vi "svx_Multitone Generator.vi"(5 "amplitude":dbl=-1.0 format="%.2f", 6 "sampling info":cluster{"Fs":dbl, "#s":dbl}={"Fs"=1000.0, "#s"=1000.0} {"#s" format="%.2p"; "Fs" format="%.2p"}, 8 "error in (no error)":errorcluster, 9 "tone phases":dbl[](array[numeric])=[137.63, 330.58, 66.37, 291.58, 225.38] format="%.2f", 10 "tone amplitudes":dbl[](array[numeric])=[1.0, 1.0, 1.0, 1.0, 1.0] format="%.2f", 11 "tone frequencies":dbl[](array[numeric])=[100.0, 200.0, 300.0, 400.0, 500.0] format="%.2f") -> (0 "error out":errorcluster, 2 "crest factor":dbl format="%.2f", 3 "signal out":waveform(dbl))   [LabVIEW 2017]
doc: "This VI generates a waveform that is the sum of integer cycle sine tones. The frequency domain representation of this waveform is a sequence of impulses at the specified tone frequencies and zero at all other frequencies. The number of tones is determined by the size of the array inputs (<B>tone frequencies</B>, <B>tone amplitudes</B>, and <B>phases</B>). First, the sine tones are generated using the frequency, phase, amplitude and samples information. This raw array is then scaled so that the largest absolute value is equal to the <B>amplitude</B> input. Finally the waveform is bundled. The X0 element of the waveform is always set equal to 0 and the delta X element is set equal to 1/(Sampling Rate)."
uses:
  <vilib>/Analysis/2dsp.llb/Inverse Real FFT.vi
  <vilib>/Analysis/5stat.llb/RMS (DBL).vi
  <vilib>/measure/NI_MABase.lvlib
  <vilib>/measure/NI_MAPro.lvlib
  <vilib>/Analysis/NI_AALPro.lvlib
  <vilib>/Analysis/NI_AALBase.lvlib
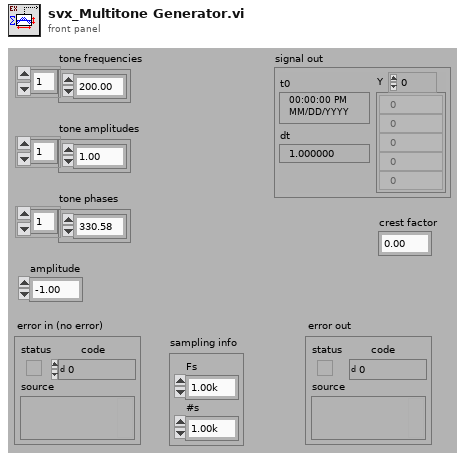
[diagram p1: front panel]
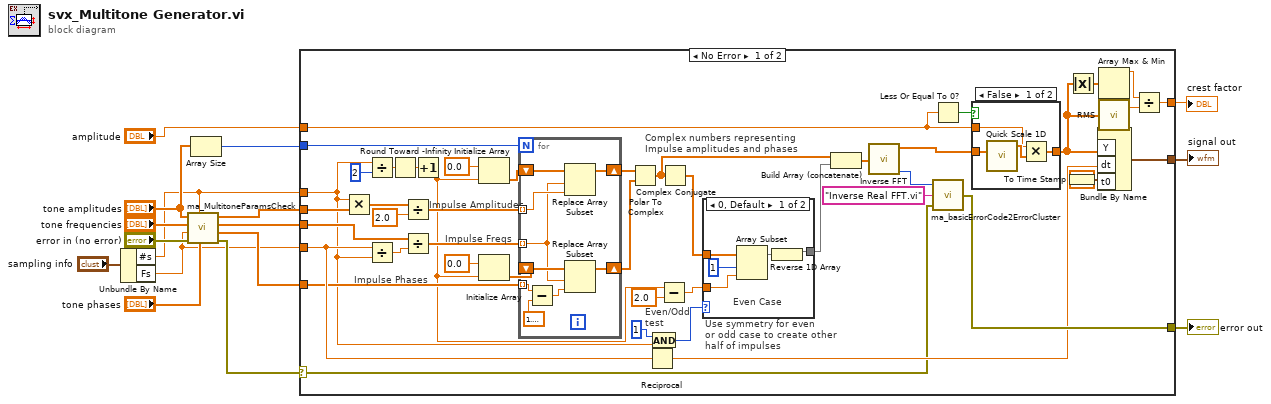
[diagram p0: block diagram]
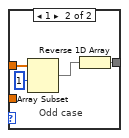
[diagram p3: hidden frame]
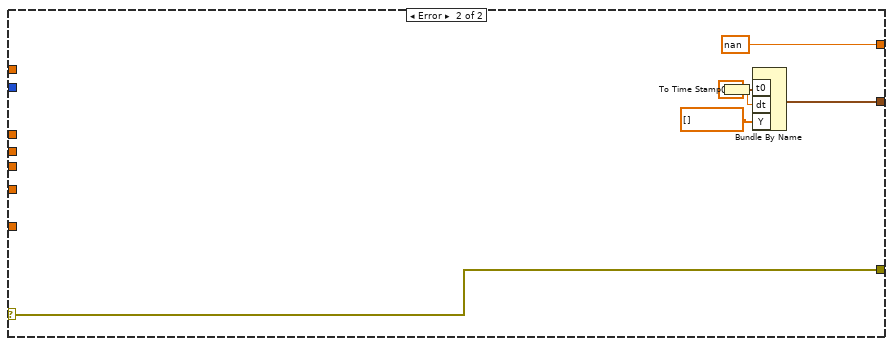
[diagram p4: hidden frame]
diagram:
  n1 = Unbundle By Name("sampling info") -> ("#s"=w4:dbl, "Fs"=w5:dbl)
  n2 = call <vilib>:"ma_MultitoneParamsCheck.vi"("Phases"="tone phases", "Samples"=w4, "error in (no error)"="error in (no error)", "Sampling Rate"=w5, "Tone Frequencies"="tone frequencies", "Tone Amplitudes"="tone amplitudes") -> ("error out"=w7:errorcluster, "Phases out"=w11:dbl[], "Tone Frequencies out"=w13:dbl[], "Tone Amplitudes out"=w8:dbl[])  [unwired: 2 in]
  n3 = Array Size(array="tone amplitudes") -> (size(s)=w15:i32)
  n4 = case shown="No Error" w7 {
    selector: w7 -> [w18 w86]
    tunnel: w5 -> [w59 _]
    tunnel: [w61 w86] -> w16
    tunnel: w15 -> [w60 _]
    tunnel: w4 -> [w32 _]
    tunnel: w13 -> [w58 _]
    tunnel: w11 -> [w37 _]
    tunnel: w8 -> [w36 _]
    tunnel: "amplitude" -> [w33 _]
    tunnel: [w25 nan] -> w2
    tunnel: [w24 w87] -> w1
    frame No Error {
      # "Impulse Phases"
      # "Use symmetry for even\nor odd case to create other\nhalf of impulses"
      # "Even/Odd\ntest"
      # "Complex numbers representing \nImpulse amplitudes and phases"
      # "Impulse Freqs"
      # "Impulse Amplitudes"
      n5 = Multiply(x=w32, y=w36) -> (x*y=w53:dbl[])
      n6 = Divide(x=w32, y=2) -> (x/y=w23:dbl)
      n7 = Divide(x=w59, y=w32) -> (x/y=w52:dbl)
      n8 = Round Toward -Infinity(1:w23) -> (0:w22:dbl)
      n9 = Divide(x=w53, y=2.0) -> (x/y=w55:dbl[])
      n10 = Divide(x=w58, y=w52) -> (x/y=w56:dbl[])
      n11 = Increment(x=w22) -> (x+1=w20:dbl)
      n12 = Initialize Array(0.0 ("Element Data"), w20) -> (w48:dbl[])
      n13 = Initialize Array(0.0 ("Element Data"), w20) -> (w47:dbl[])
      n14 = for {
        N: w60 -> [_]
        tunnel: w56 -> [w79] mode=indexing
        tunnel: w55 -> [w84] mode=indexing
        shift-right: [w82] -> w45
        shift-left: w48 -> [w83]
        shift-right: [w81] -> w46
        shift-left: w47 -> [w80]
        tunnel: w37 -> [w77] mode=indexing
        n15 = Subtract(x=w77, y=1.5707963267948966) -> (x-y=w78:dbl)
        n16 = Replace Array Subset(array=w83, new element=w84, index=w79) -> (w82:dbl[])
        n17 = Replace Array Subset(array=w80, new element=w78, index=w79) -> (w81:dbl[])
      }
      n18 = Polar To Complex(1:w46, 2:w45) -> (0:w44:cdb[])
      n19 = Reciprocal(x=w59) -> (1/x=w31:dbl)
      n20 = And(x=1, y=w32) -> (x .and. y?=w43:i32)
      n21 = Subtract(x=w20, y=2.0) -> (x-y=w21:dbl)
      n22 = Complex Conjugate(1:w44) -> (0:w42:cdb[])
      n23 = case shown="0, Default" w43 {
        tunnel: [w71 w72] -> w40
        tunnel: w42 -> [w70 w75]
        tunnel: w21 -> [w67 _]
        frame 0, Default {
          # "Even Case"
          n24 = Array Subset(array=w70, index=1 ("Array Index"), length=w67) -> (w69:cdb[])
          n25 = Reverse 1D Array(array=w69) -> (reversed array=w71:cdb[])
        }
        frame 1 {
          # "Odd case"
          n26 = Array Subset(array=w75, index=1 ("Array Index")) -> (w73:cdb[])  [unwired: 1 in]
          n27 = Reverse 1D Array(array=w73) -> (reversed array=w72:cdb[])
        }
      }
      n28 = Build Array (concatenate)(w44, w40) -> (w41:cdb[])
      n29 = call-poly <vilib>:"Inverse FFT.vi"("FFT {X}"=w41) -> ("error"=w39:i32, "X"=w35:dbl[])  [unwired: 9 in]
      n30 = Less Or Equal To 0?(x=w33) -> (x <= 0?=w34:bool)
      n31 = call <vilib>:"ma_basicErrorCode2ErrorCluster.vi"("error in (no error)"=w18, "subVI name"="Inverse Real FFT.vi" ("subVI Name"), "Error Code"=w39) -> ("error out"=w61:errorcluster)
      n32 = case shown="False" w34 {
        tunnel: w35 -> [w65 w66]
        tunnel: [w64 w66] -> w28
        tunnel: w33 -> [w62 _]
        frame False {
          n33 = call <vilib>:"Quick Scale 1D.vi"("X"=w65) -> ("Y[i]=X[i]/Max|X|"=w63:dbl[])  [unwired: 2 out]
          n34 = Multiply(x=w62, y=w63) -> (x*y=w64:dbl[])
        }
        frame True {
        }
      }
      n35 = To Time Stamp(1:0.0 ("Waveform Component")) -> (0:w17:timestamp)
      n36 = Absolute Value(x=w28) -> (abs(x)=w29:dbl[])
      n37 = Bundle By Name("Y"=w28, "dt"=w31, "t0"=w17) -> (w24:waveform(dbl))  [unwired: 1 in]
      n38 = Array Max & Min(array=w29) -> (max value=w27:dbl)  [unwired: 3 out]
      n39 = call-poly <vilib>:"RMS.vi"("X"=w28) -> ("rms value"=w26:dbl)  [unwired: 1 out]
      n40 = Divide(x=w27, y=w26) -> (x/y=w25:dbl)
    }
    frame Error {
      w89 = 0.0 ("t0")
      n41 = To Time Stamp(1:w89) -> (0:w85:timestamp)
      n42 = Bundle By Name("t0"=w85, "dt"=w89, "Y"=dbl[] []) -> (w87:waveform(dbl))  [unwired: 1 in]
    }
  }
  "error out" <- w16
  "signal out" <- w1
  "crest factor" <- w2
